vi "Verify.vi"(7 "Actor":refnum<class "Actor.lvclass">) -> (3 "Stats":T1)   [LabVIEW 2020, in "jettl.lvlib" / "Actor.lvclass"]
uses:
  Actor.lvclass
  MsgNames.ctl
  jettl.lvlib
  Stats.ctl
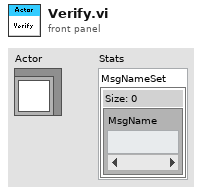
[diagram p1: front panel]
types:
  T1 = typedef "jettl.lvlib/Stats.ctl" = cluster{"MsgNameSet":T2}
  T2 = typedef "jettl.lvlib/MsgNames.ctl" = set{string}
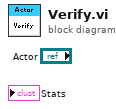
[diagram p0: block diagram]
diagram:
